vi "PTP Slave.vi"() -> ()   [LabVIEW 8.6]
uses:
  <libdir>/resource/objmgr/UeiDaq.rc
panel:
  out "PTP Time Stamp":timestamp
  out "PTP UTC Time":cluster{"Seconds":u32, "Nanoseconds":u32}
  out "Array":T1(array[cluster]) {"Grand Master Clock ID" format="%x"; "Master Clock ID" format="%x"}
  in  "stop":bool
  out "Locked":bool[](array[boolean])
  in  "Sampling rate":dbl
  in  "CPU Sync Resources":string[](array[string])
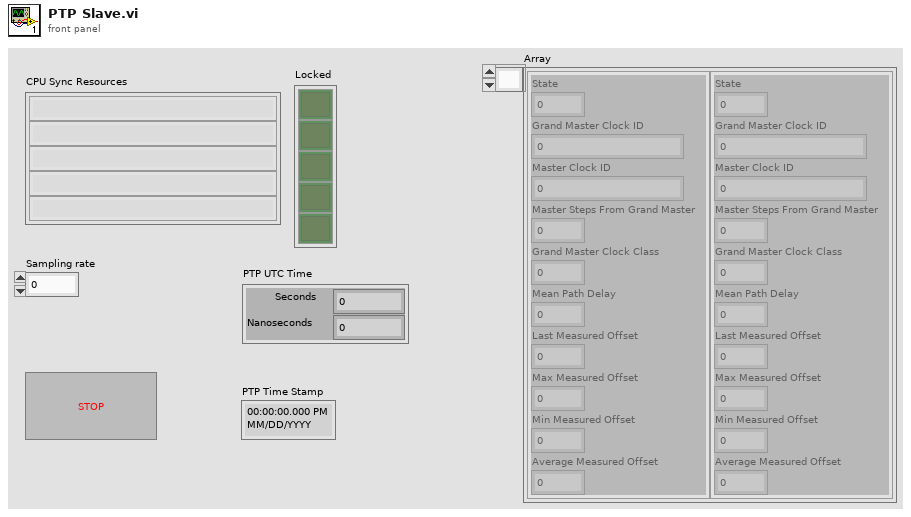
[diagram p1: front panel]
types:
  T1 = cluster{"State":u16, "Grand Master Clock ID":u64, "Master Clock ID":u64, "Master Steps From Grand Master":u32, "Grand Master Clock Class":u32, "Mean Path Delay":i32, "Last Measured Offset":i32, "Max Measured Offset":i32, "Min Measured Offset":i32, "Average Measured Offset":i32}[]
  T2 = cluster{"State":u16, "Grand Master Clock ID":u64, "Master Clock ID":u64, "Master Steps From Grand Master":u32, "Grand Master Clock Class":u32, "Mean Path Delay":i32, "Last Measured Offset":i32, "Max Measured Offset":i32, "Min Measured Offset":i32, "Average Measured Offset":i32}
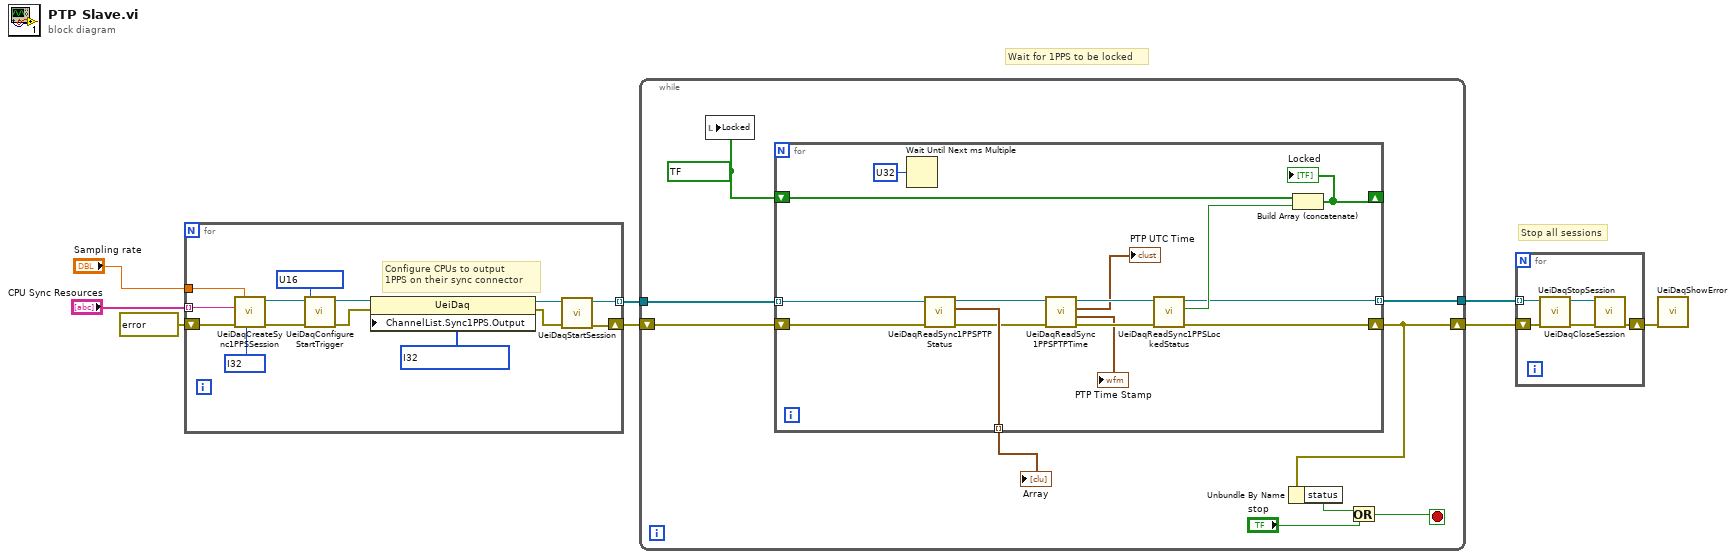
[diagram p0: block diagram]
diagram:
  # "Stop all sessions"
  # "Wait for 1PPS to be locked"
  n1 = for {
    shift-right: [w15] -> w5
    shift-left: errorcluster ? ("error out") -> [w22]
    tunnel: "CPU Sync Resources" -> [w21] mode=indexing
    tunnel: "Sampling rate" -> [w20]
    tunnel: [w14] -> w4 mode=indexing
    w13 = u16 ? items=["Immediate", "Software", "External", "Signal", "Next1PPS"] ("Trigger source")
    w18 = i32[] ? items=["None", "Output0", "Output1"] ("Channel List:Sync 1PPS:Output")
    w19 = i32 ? items=["Clock", "1588", "NTP", "IRIG"] ("Mode")
    # "Configure CPUs to output\n1PPS on their sync connector"
    n2 = call "UeiDaqCreateSync1PPSSession.vi"("Mode"=w19, "Output Rate"=w20, "error in (no error)"=w22, "Resource"=w21) -> ("error out"=w11:errorcluster, "UeiDaq Refnum Out"=w12:refnum<k20>)  [unwired: 2 in, 4 out]
    n3 = call "UeiDaqConfigureStartTrigger.vi"("error in (no error)"=w11, "Trigger source"=w13, "UeiDaq Refnum In"=w12) -> ("error out"=w9:errorcluster, "UeiDaq Refnum Out"=w10:refnum<k20>)  [unwired: 1 in, 6 out]
    n4 = property class="UeiDaq"(reference=w10, error in=w9, "ChannelList.Sync1PPS.Output"=w18) -> (reference out=w17:refnum<k20>, error out=w16:errorcluster)
    n5 = call "UeiDaqStartSession.vi"("error in (no error)"=w16, "UeiDaq Refnum In"=w17) -> ("error out"=w15:errorcluster, "UeiDaq Refnum Out"=w14:refnum<k20>)  [unwired: 8 out]
  }
  n6 = while {
    shift-right: [w25] -> w2
    shift-left: w5 -> [w29]
    tunnel: w4 -> [w28]
    tunnel: [w27] -> w1
    stop <- w26 stop-if-true
    w31 = bool[] ? ("Locked")
    n7 = local write "Locked"(w31) -> ()
    n8 = for {
      shift-right: [w42] -> w25
      shift-left: w29 -> [w39]
      shift-right: [w45] -> _
      shift-left: w31 -> [w46]
      tunnel: [w41] -> w27 mode=indexing
      tunnel: w28 -> [w40] mode=indexing
      tunnel: [w38] -> w23 mode=indexing
      n9 = Wait Until Next ms Multiple(millisecond multiple=u32 ?) -> ()  [unwired: 1 out]
      n10 = call "UeiDaqReadSync1PPSPTPStatus.vi"("error in (no error)"=w39, "UeiDaq Refnum In"=w40) -> ("error out"=w35:errorcluster, "PTP Status"=w38:T2, "UeiDaq Refnum Out"=w37:refnum<k20>)  [unwired: 7 out]
      n11 = call "UeiDaqReadSync1PPSPTPTime.vi"("error in (no error)"=w35, "UeiDaq Refnum In"=w37) -> ("error out"=w34:errorcluster, "Time Stamp"=→"PTP Time Stamp":timestamp, "PTP Time"=→"PTP UTC Time":cluster{"Seconds":u32, "Nanoseconds":u32}, "UeiDaq Refnum Out"=w36:refnum<k20>)  [unwired: 6 in]
      n12 = call "UeiDaqReadSync1PPSLockedStatus.vi"("error in (no error)"=w34, "UeiDaq Refnum In"=w36) -> ("error out"=w42:errorcluster, "Locked"=w43:bool, "UeiDaq Refnum Out"=w41:refnum<k20>)  [unwired: 7 in]
      n13 = Build Array (concatenate)(w46, w43) -> (w45:bool[])
      "Locked" <- w45
    }
    "Array" <- w23
    n14 = Unbundle By Name(w25) -> ("status"=w30:bool)
    n15 = Or(x=w30, y="stop") -> (x .or. y?=w26:bool)
  }
  n16 = for {
    tunnel: w1 -> [w47] mode=indexing
    shift-right: [w51] -> w3
    shift-left: w2 -> [w49]
    tunnel: [w47] -> _ mode=indexing
    n17 = call "UeiDaqStopSession.vi"("error in (no error)"=w49, "UeiDaq Refnum In"=w47) -> ("error out"=w48:errorcluster, "UeiDaq Refnum Out"=w50:refnum<k20>)  [unwired: 8 out]
    n18 = call "UeiDaqCloseSession.vi"("error in (no error)"=w48, "UeiDaq Refnum In"=w50) -> ("error out"=w51:errorcluster)  [unwired: 1 in, 8 out]
  }
  n19 = call "UeiDaqShowError.vi"("error in (no error)"=w3) -> ()  [unwired: 2 in, 9 out]
